vi "Octaves Enum to Ratio.vi"(11 "octaves":T1(ring)=enum."1/3") -> (3 "ratio":dbl=nan)   [LabVIEW 2017, in "Octave with Cursors.xctl"]
uses:
  <vilib>/addons/_XControls/Octave with Cursors/Octave with Cursors.xctl
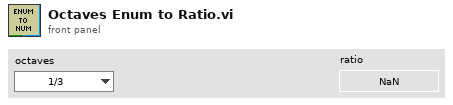
[diagram p1: front panel]
types:
  T1 = enum16{"Free", "1/24", "1/12", "1/6", "1/3", "1", "2", "4", "6", "8", "10"}
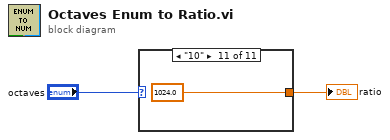
[diagram p0: block diagram]
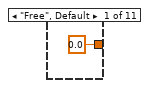
[diagram p2: hidden frame]
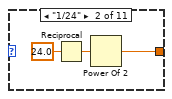
[diagram p3: hidden frame]
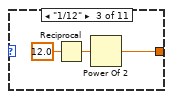
[diagram p4: hidden frame]
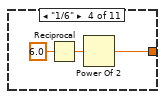
[diagram p5: hidden frame]
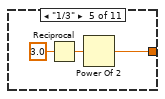
[diagram p6: hidden frame]
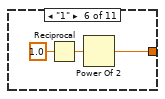
[diagram p7: hidden frame]
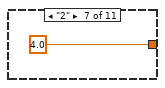
[diagram p8: hidden frame]
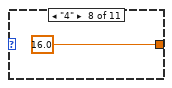
[diagram p9: hidden frame]
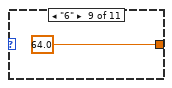
[diagram p10: hidden frame]
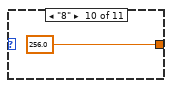
[diagram p11: hidden frame]
diagram:
  n1 = case shown="\"10\"" "octaves" {
    tunnel: [0.0 w4 w7 w10 w13 w16 4.0 ("Fixed ratio (octaves)") 16.0 ("Fixed ratio (octaves)") 64.0 ("Fixed ratio (octaves)") 256.0 ("Fixed ratio (octaves)") 1024.0 ("Fixed ratio (octaves)")] -> w1
    frame "Free", Default {
    }
    frame "1/24" {
      n2 = Reciprocal(x=24.0 ("Fixed ratio (octaves)")) -> (1/x=w5:dbl)
      n3 = Power Of 2(x=w5) -> (2^x=w4:dbl)
    }
    frame "1/12" {
      n4 = Reciprocal(x=12.0 ("Fixed ratio (octaves)")) -> (1/x=w8:dbl)
      n5 = Power Of 2(x=w8) -> (2^x=w7:dbl)
    }
    frame "1/6" {
      n6 = Reciprocal(x=6.0 ("Fixed ratio (octaves)")) -> (1/x=w11:dbl)
      n7 = Power Of 2(x=w11) -> (2^x=w10:dbl)
    }
    frame "1/3" {
      n8 = Reciprocal(x=3.0 ("Fixed ratio (octaves)")) -> (1/x=w14:dbl)
      n9 = Power Of 2(x=w14) -> (2^x=w13:dbl)
    }
    frame "1" {
      n10 = Reciprocal(x=1.0 ("Fixed ratio (octaves)")) -> (1/x=w17:dbl)
      n11 = Power Of 2(x=w17) -> (2^x=w16:dbl)
    }
    frame "2" {
    }
    frame "4" {
    }
    frame "6" {
    }
    frame "8" {
    }
    frame "10" {
    }
  }
  "ratio" <- w1
